vi "Configure Modulation.vi"   [LabVIEW 2012, in "RIGOL DG4000 Series.lvlib"]
doc: "Configure Modulation polymorphic VI."
uses:
  <instrlib>/RIGOL DG4000 Series/RIGOL DG4000 Series.lvlib
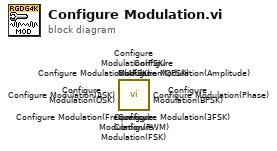
[diagram p0: block diagram]
diagram:
  n1 = call <instrlib>:"Configure Modulation(PWM).vi"() -> ()  [unwired: 14 in, 2 out]
  n2 = call <instrlib>:"Configure Modulation(QPSK).vi"() -> ()  [unwired: 14 in, 2 out]
  n3 = call <instrlib>:"Configure Modulation(OSK).vi"() -> ()  [unwired: 14 in, 2 out]
  n4 = call <instrlib>:"Configure Modulation(BPSK).vi"() -> ()  [unwired: 14 in, 2 out]
  n5 = call <instrlib>:"Configure Modulation(4FSK).vi"() -> ()  [unwired: 14 in, 2 out]
  n6 = call <instrlib>:"Configure Modulation(3FSK).vi"() -> ()  [unwired: 14 in, 2 out]
  n7 = call <instrlib>:"Configure Modulation(PSK).vi"() -> ()  [unwired: 14 in, 2 out]
  n8 = call <instrlib>:"Configure Modulation(FSK).vi"() -> ()  [unwired: 14 in, 2 out]
  n9 = call <instrlib>:"Configure Modulation(ASK).vi"() -> ()  [unwired: 14 in, 2 out]
  n10 = call <instrlib>:"Configure Modulation(Phase).vi"() -> ()  [unwired: 14 in, 2 out]
  n11 = call <instrlib>:"Configure Modulation(Frequency).vi"() -> ()  [unwired: 14 in, 2 out]
  n12 = call <instrlib>:"Configure Modulation(Amplitude).vi"() -> ()  [unwired: 14 in, 2 out]
